vi "provide_OME_data.vi"(8 "error in (no error)":errorcluster, 9 "parameters":T1, 10 "OME XMLElement in":refnum<class "XMLElement.lvclass">, 11 "ImageCollection in":refnum<class "ImageCollection.lvclass">) -> (0 "error out":errorcluster, 2 "OME XMLElement out":refnum<class "XMLElement.lvclass">, 3 "ImageCollection out":refnum<class "ImageCollection.lvclass">)   [LabVIEW 2010, in "ImageCollection.lvclass"]
uses:
  ImageCollection.lvclass
  OME_parameters_cluster.ctl
  dimension_order_enum.ctl
  XMLElement/XMLElement/XMLElement.lvclass
  enumerations/unit.ctl
  ImageCollection.lvclass/ImageCollection.ctl
  Image/Image/Image.lvclass
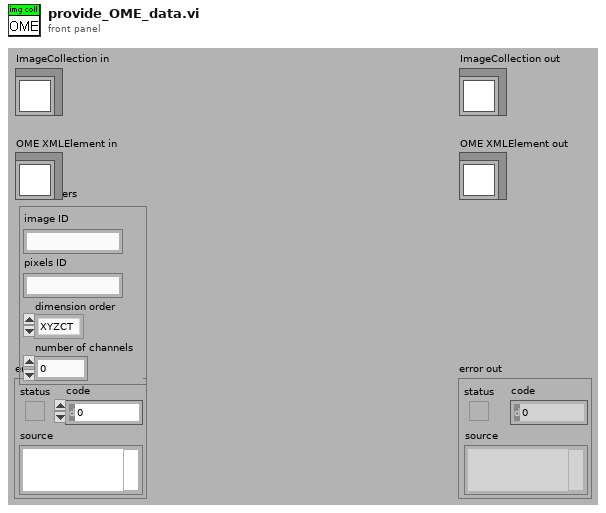
[diagram p1: front panel]
types:
  T1 = typedef "OME_parameters_cluster.ctl" = cluster{"image ID":string, "pixels ID":string, "dimension order":T2, "number of channels":i32}
  T2 = typedef "dimension_order_enum.ctl" = enum16{"XYZCT", "XYZTC", "XYCTZ", "XYCZT", "XYTCZ", "XYTZC"}
  T3 = typedef "Image.lvclass/unit.ctl" = enum16{"um", "s"}
  T4 = typedef "type_enum.ctl" = enum16{"undefined", "movie", "z-stack"}
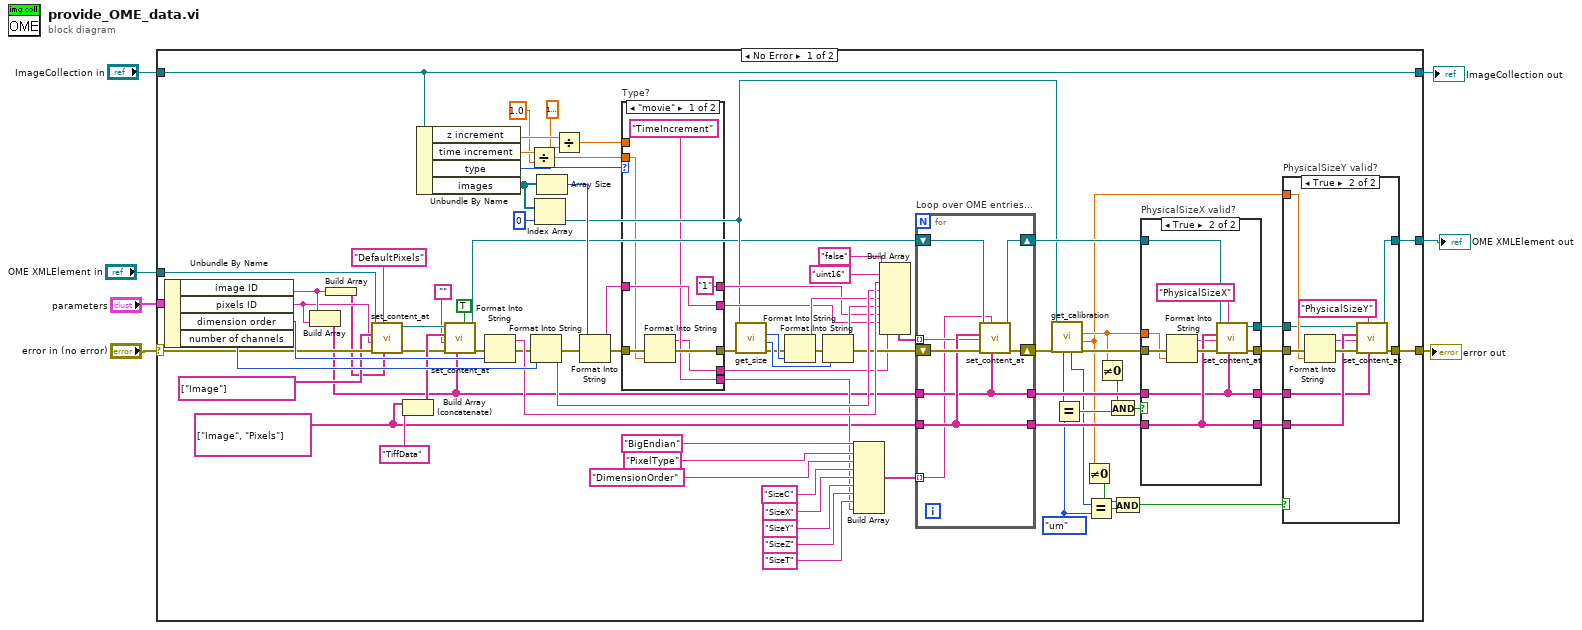
[diagram p0: block diagram]
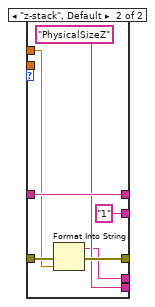
[diagram p4: hidden frame]
diagram:
  n1 = case shown="No Error" "error in (no error)" {
    selector: "error in (no error)" -> [w20 w142]
    tunnel: [w56 w142] -> w6
    tunnel: [w88 w141] -> w4
    tunnel: "ImageCollection in" -> [w88 w141]
    tunnel: "OME XMLElement in" -> [w18 w140]
    tunnel: [w53 w140] -> w1
    tunnel: "parameters" -> [w91 _]
    frame No Error {
      w15 = string[] ["Image", "Pixels"] ("key array")
      w42 = unit."um" ("y")
      n2 = Unbundle By Name(w91) -> ("image ID"=w14:string, "pixels ID"=w12:string, "dimension order"=w90:T2, "number of channels"=w89:i32)
      n3 = Build Array(w14, w12) -> (w11:string[])
      n4 = Build Array(w14) -> (w9:string[])
      n5 = call "set_content_at.vi"("id chain"=w9, "attribute name"="DefaultPixels", "error in (no error)"=w20, "content"=w12, "key chain"=string[] ["Image"] ("key array"), "Element in"=w18) -> ("error out"=w19:errorcluster, "Element out"=w17:refnum<class "XMLElement.lvclass">)  [unwired: 4 in]
      n6 = Build Array (concatenate)(w15, "TiffData") -> (w22:string[])
      n7 = Unbundle By Name(w88) -> ("z increment"=w36:dbl[unit], "time increment"=w33:dbl[unit], "type"=w68:T4, "images"=w71:refnum<class "Image.lvclass">[])
      n8 = call "set_content_at.vi"("enforce empty content?"=TRUE, "id chain"=w11, "error in (no error)"=w19, "content"="", "key chain"=w22, "Element in"=w17) -> ("error out"=w24:errorcluster, "Element out"=w21:refnum<class "XMLElement.lvclass">)  [unwired: 4 in]
      n9 = Format Into String(error in=w24, w90) -> (resulting string=w85:string, error out=w81:errorcluster)  [unwired: 2 in]
      n10 = Divide(x=w33, y=dbl[unit] 1.0) -> (x/y=w32:dbl)
      n11 = Format Into String(error in=w81, w89) -> (resulting string=w80:string, error out=w30:errorcluster)  [unwired: 2 in]
      n12 = Index Array(array=w71, index=0) -> (element=w48:refnum<class "Image.lvclass">)
      n13 = Array Size(array=w71) -> (size(s)=w67:i32)
      n14 = Divide(x=w36, y=dbl[unit] 1e-06) -> (x/y=w34:dbl)
      n15 = Format Into String(error in=w30, w67) -> (resulting string=w65:string, error out=w27:errorcluster)  [unwired: 2 in]
      n16 = case "Type?" shown="\"movie\"" w68 {
        tunnel: w65 -> [w124 w131]
        tunnel: ["1" w131] -> w64
        tunnel: [w124 "1"] -> w63
        tunnel: w34 -> [_ w127]
        tunnel: w32 -> [w120 _]
        tunnel: w27 -> [w122 w129]
        tunnel: [w121 w128] -> w28
        tunnel: ["TimeIncrement" ("String") "PhysicalSizeZ"] -> w26
        tunnel: [w118 w125] -> w25
        frame "movie" {
          n17 = Format Into String(error in=w122, w120) -> (resulting string=w118:string, error out=w121:errorcluster)  [unwired: 2 in]
        }
        frame "z-stack", Default {
          n18 = Format Into String(error in=w129, w127) -> (resulting string=w125:string, error out=w128:errorcluster)  [unwired: 2 in]
        }
      }
      n19 = call-dynamic "get_size.vi"("error in (no error)"=w28, "Image in"=w48) -> ("error out"=w29:errorcluster, "y resolution"=w62:i32, "x resolution"=w61:i32)  [unwired: 2 in, 5 out]
      n20 = Format Into String(error in=w29, w61) -> (resulting string=w77:string, error out=w78:errorcluster)  [unwired: 2 in]
      n21 = Format Into String(error in=w78, w62) -> (resulting string=w76:string, error out=w60:errorcluster)  [unwired: 2 in]
      n22 = Build Array("BigEndian" ("String"), "PixelType" ("String"), "DimensionOrder" ("String"), "SizeC" ("String"), "SizeX" ("String"), "SizeY" ("String"), "SizeZ" ("String"), "SizeT" ("String"), w26) -> (w73:string[])
      n23 = Build Array("false", "uint16", w85, w80, w77, w76, w64, w63, w25) -> (w72:string[])
      n24 = for "Loop over OME entries..." {
        shift-right: [w138] -> w59
        shift-left: w60 -> [w139]
        tunnel: w73 -> [w132] mode=indexing
        tunnel: w72 -> [w134] mode=indexing
        tunnel: w11 -> [w133]
        tunnel: w15 -> [w135]
        shift-right: [w136] -> w54
        shift-left: w21 -> [w137]
        tunnel: [w135] -> w52
        tunnel: [w133] -> w51
        n25 = call "set_content_at.vi"("id chain"=w133, "attribute name"=w132, "error in (no error)"=w139, "content"=w134, "key chain"=w135, "Element in"=w137) -> ("error out"=w138:errorcluster, "Element out"=w136:refnum<class "XMLElement.lvclass">)  [unwired: 4 in]
      }
      n26 = call "get_calibration.vi"("error in (no error)"=w59, "Image.lvclass in"=w48) -> ("error out"=w58:errorcluster, "y"=w37:dbl, "x"=w38:dbl, "y unit"=w43:T3, "x unit"=w47:T3)  [unwired: 2 in, 3 out]
      n27 = Equal?(x=w47, y=w42) -> (x = y?=w46:bool)
      n28 = Not Equal To 0?(x=w37) -> (x != 0?=w39:bool)
      n29 = Equal?(x=w43, y=w42) -> (x = y?=w41:bool)
      n30 = Not Equal To 0?(x=w38) -> (x != 0?=w45:bool)
      n31 = And(x=w45, y=w46) -> (x .and. y?=w44:bool)
      n32 = And(x=w39, y=w41) -> (x .and. y?=w40:bool)
      n33 = case "PhysicalSizeX valid?" shown="True" w44 {
        tunnel: w58 -> [w104 w117]
        tunnel: [w104 w114] -> w57
        tunnel: [w105 w113] -> w55
        tunnel: w54 -> [w105 w112]
        tunnel: w52 -> [w106 w111]
        tunnel: w51 -> [w107 w109]
        tunnel: [w107 w109] -> w50
        tunnel: [w106 w111] -> w49
        tunnel: w38 -> [_ w116]
        frame False {
        }
        frame True {
          n34 = Format Into String(error in=w117, w116) -> (resulting string=w110:string, error out=w115:errorcluster)  [unwired: 2 in]
          n35 = call "set_content_at.vi"("id chain"=w109, "attribute name"="PhysicalSizeX" ("String"), "error in (no error)"=w115, "content"=w110, "key chain"=w111, "Element in"=w112) -> ("error out"=w114:errorcluster, "Element out"=w113:refnum<class "XMLElement.lvclass">)  [unwired: 4 in]
        }
      }
      n36 = case "PhysicalSizeY valid?" shown="True" w40 {
        tunnel: w57 -> [w93 w103]
        tunnel: [w93 w100] -> w56
        tunnel: w55 -> [w92 w98]
        tunnel: [w92 w97] -> w53
        tunnel: w50 -> [_ w95]
        tunnel: w49 -> [_ w99]
        tunnel: w37 -> [_ w102]
        frame False {
        }
        frame True {
          n37 = Format Into String(error in=w103, w102) -> (resulting string=w96:string, error out=w101:errorcluster)  [unwired: 2 in]
          n38 = call "set_content_at.vi"("id chain"=w95, "attribute name"="PhysicalSizeY" ("String"), "error in (no error)"=w101, "content"=w96, "key chain"=w99, "Element in"=w98) -> ("error out"=w100:errorcluster, "Element out"=w97:refnum<class "XMLElement.lvclass">)  [unwired: 4 in]
        }
      }
    }
    frame Error {
    }
  }
  "error out" <- w6
  "ImageCollection out" <- w4
  "OME XMLElement out" <- w1
